vi "Store Metadata in TDMS.vi"(5 "Value":variant, 7 "name":string, 8 "Error In":errorcluster, 9 "channel name":string, 10 "group name":string, 11 "tdms file":refnum<k34>) -> (0 "Error Out":errorcluster, 1 "channel name out":string, 2 "group name out":string, 3 "tdms file out":refnum<k34>)   [LabVIEW 2016]
uses:
  <vilib>/Utility/Data Type/Type Definitions/Data Type.ctl
  <vilib>/Utility/Data Type/NI_Data Type.lvlib
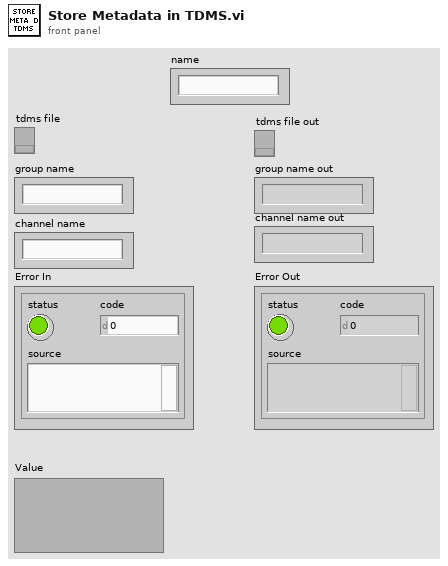
[diagram p1: front panel]
types:
  T1 = typedef "NI_Data Type.lvlib/Data Type.ctl" = enum8{"Invalid Type", "Void", "I8", "I16", "I32", "I64", "U8", "U16", "U32", "U64", "Single Float", "Double Float", "Extended Float", "Single Complex", "Double Complex", "Extended Complex", "Enum U8", "Enum U16", "Enum U32", "Enum U64", "Single Float With Unit", "Double Float With Unit", "Extended Float With Unit", "Single Complex with Unit", "Double Complex with Unit", "Extended Complex with Unit", "Boolean", "String", "Path", "Picture", "Tag", "Array", "Cluster", "Variant", "LV Variant", "Waveform", "Timestamp", "Digital Waveform", "Digital Data", "ExpressData", "Refnum", "External Data", "VI", "Poly VI", "LabVIEW Class Instance", "Fixed Point"}
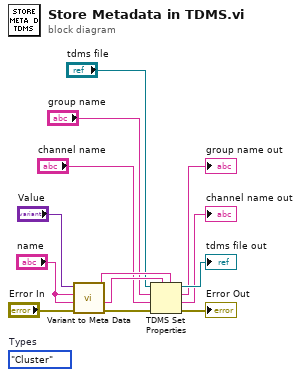
[diagram p0: block diagram]
diagram:
  (unwired) Data_Type."Cluster"  # Types
  n1 = call "Variant to Meta Data.vi"("Error In"="Error In", "Name"="name", "key (optional)"="name", "Value"="Value") -> ("Error Out"=w8:errorcluster, "Name out"=w9:string, "Meta data"=w10:string)  [unwired: 4 in, 1 out]
  n2 = TDMS Set Properties(5:w10, 7:w9, 8:w8, 9:"channel name", 10:"group name", 11:"tdms file") -> (0:→"Error Out":errorcluster, 1:→"channel name out":string, 2:→"group name out":string, 3:→"tdms file out":refnum<k34>)
